vi "Device.vi"(8 "error in (no error)":errorcluster, 11 "Node Ptr":T1 format="%.0x") -> (0 "error out":errorcluster)   [LabVIEW 2013]
uses:
  <vilib>/NI Veristand/Custom Device API/Custom Device Item Ref.ctl
  <vilib>/NI Veristand/Custom Device API/Custom Device API.lvlib
panel:
  in  "Header":cluster{"Section Name":string}={"Section Name"="Custom Device Item Settings"}
  in  "Description":string
  in  "Name":string
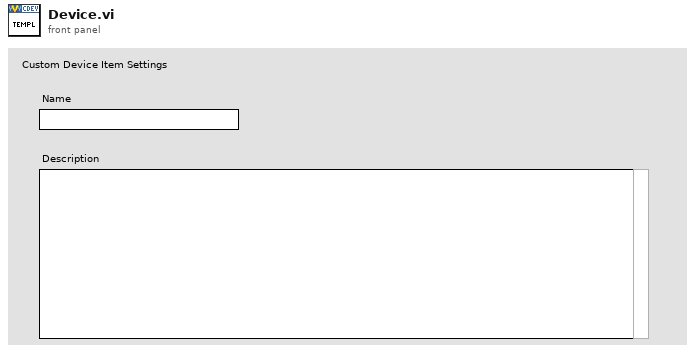
[diagram p1: front panel]
types:
  T1 = typedef "Custom Device API.lvlib/Custom Device Item Ref.ctl" = u64
  T2 = typedef "Custom Device API.lvlib/Custom Device Item Info.ctl" = cluster{"Name":string, "Is Channel":bool, "GUID":string, "Is Waveform":bool}
  T3 = typedef "Custom Device API.lvlib/Custom Device Commands.ctl" = enum16{"Default", "Item renamed", "Shutdown", "Dynamic button pressed"}
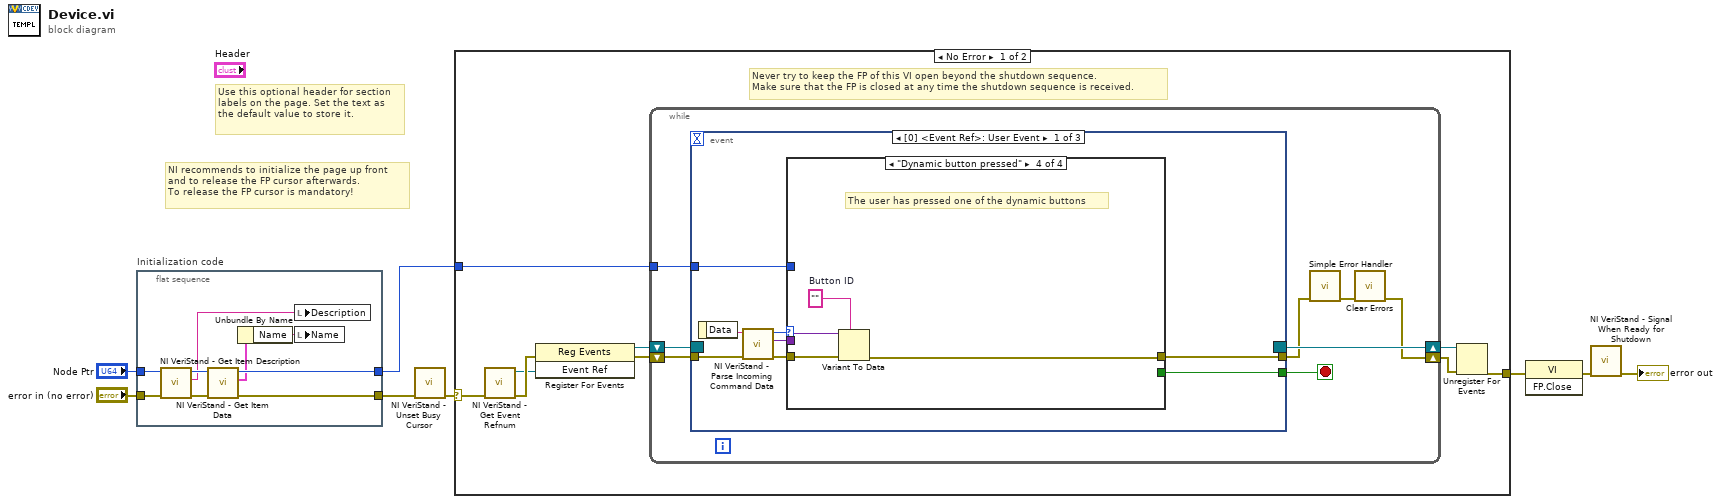
[diagram p0: block diagram]
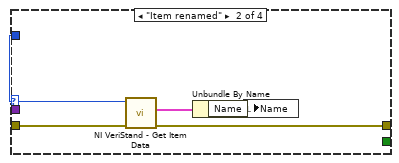
[diagram p3: hidden frame]
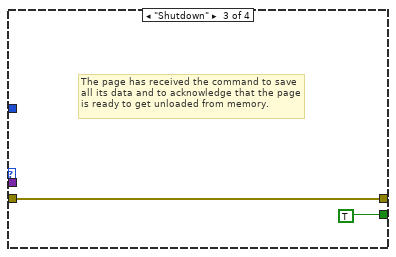
[diagram p4: hidden frame]
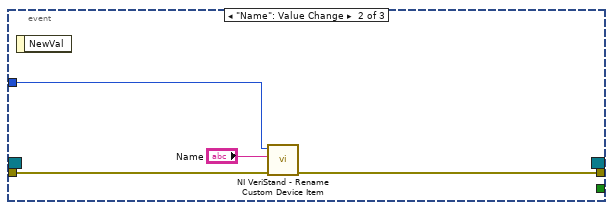
[diagram p5: hidden frame]
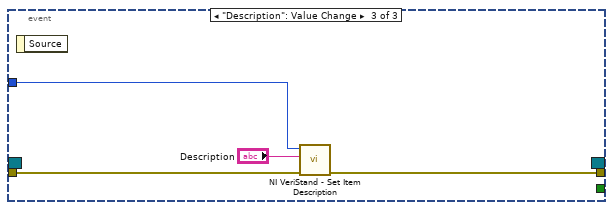
[diagram p6: hidden frame]
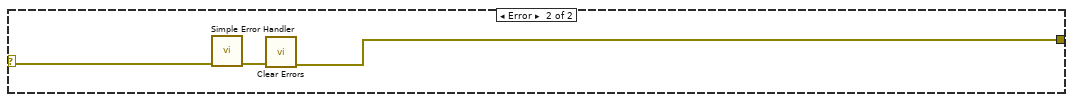
[diagram p7: hidden frame]
diagram:
  # "Use this optional header for section labels on the page. Set the text as the default value to store it."
  # "NI recommends to initialize the page up front\nand to release the FP cursor afterwards.\nTo release the FP cursor is mandatory!"
  n1 = flat-sequence "Initialization code" {
    tunnel: "error in (no error)" -> [w15]
    tunnel: "Node Ptr" -> [w14]
    tunnel: [w9] -> w4
    tunnel: [w17] -> w1
    frame #0 {
      n2 = call <vilib>:"NI VeriStand - Get Item Description.vi"("error in (no error)"=w15, "Item Ref in"=w14) -> ("error out"=w12:errorcluster, "Description"=w13:string, "Item Ref out"=w16:T1)  [unwired: 7 out]
      n3 = call <vilib>:"NI VeriStand - Get Item Data.vi"("error in (no error)"=w12, "Item Ref in"=w16) -> ("error out"=w9:errorcluster, "Item Info"=w11:T2, "Item Ref out"=w17:T1)  [unwired: 7 out]
      n4 = Unbundle By Name(w11) -> ("Name"=w10:string)
      n5 = local write "Description"(w13) -> ()
      n6 = local write "Name"(w10) -> ()
    }
  }
  n7 = call <vilib>:"NI VeriStand - Unset Busy Cursor.vi"("error in (no error)"=w4) -> ("error out"=w3:errorcluster)  [unwired: 10 out]
  n8 = case shown="No Error" w3 {
    selector: w3 -> [w18 w65]
    tunnel: [w23 w63] -> w8
    tunnel: w1 -> [w19 _]
    frame No Error {
      # "Never try to keep the FP of this VI open beyond the shutdown sequence.\nMake sure that the FP is closed at any time the shutdown sequence is received."
      n9 = call <vilib>:"NI VeriStand - Get Event Refnum.vi"("error in (no error)"=w18) -> ("error out"=w26:errorcluster, "Event Ref"=w22:refnum<user-event>)  [unwired: 9 out]
      n10 = register-events(error in=w26, w22) -> (reference out=w20:refnum<event-registration>, error out=w21:errorcluster)  [unwired: 1 in]
      n11 = while {
        tunnel: w19 -> [w30]
        shift-right: [w27] -> w24
        shift-left: w21 -> [w33]
        shift-right: [w34] -> w25
        shift-left: w20 -> [w32]
        stop <- w31 stop-if-true
        n12 = event shown="[0] <Event Ref>: User Event" {
          selector: w32 -> [_ _ _]
          dyn-events: [_ _ _] -> w34
          timeout: _ -> [_ _ _]
          tunnel: w33 -> [w42 w58 w61]
          tunnel: [w38 _ _] -> w31
          tunnel: [w37 w57 w60] -> w29
          tunnel: w30 -> [w36 w56 w62]
          event User Event {
            n13 = event-data() -> ("Data"=w41:string)  [unwired: 1 out]
            n14 = call <vilib>:"NI VeriStand - Parse Incoming Command Data.vi"("error in (no error)"=w42, "Incoming data"=w41) -> ("error out"=w40:errorcluster, "Outgoing data"=w35:variant, "Action"=w39:T3)  [unwired: 7 out]
            n15 = case shown="\"Dynamic button pressed\"" w39 {
              tunnel: w40 -> [w43 w48 w49 w54]
              tunnel: [_ _ TRUE _] -> w38
              tunnel: [w43 w45 w49 w51] -> w37
              tunnel: w36 -> [_ w47 _ _]
              tunnel: w35 -> [_ _ _ w53]
              frame "Default", Default {
              }
              frame "Item renamed" {
                n16 = call <vilib>:"NI VeriStand - Get Item Data.vi"("error in (no error)"=w48, "Item Ref in"=w47) -> ("error out"=w45:errorcluster, "Item Info"=w46:T2)  [unwired: 8 out]
                n17 = Unbundle By Name(w46) -> ("Name"=w44:string)
                n18 = local write "Name"(w44) -> ()
              }
              frame "Shutdown" {
                # "The page has received the command to save all its data and to acknowledge that the page is ready to get unloaded from memory."
              }
              frame "Dynamic button pressed" {
                w52 = ""  # Button ID
                # "The user has pressed one of the dynamic buttons"
                n19 = Variant To Data(error in=w54, type=w52, Variant=w53) -> (error out=w51:errorcluster)  [unwired: 1 out]
              }
            }
          }
          event "Name": Value Change {
            n20 = event-data() -> ()  [unwired: 2 out]
            n21 = call <vilib>:"NI VeriStand - Rename Custom Device Item.vi"("error in (no error)"=w58, "New Name"="Name", "Item Ref in"=w56) -> ("error out"=w57:errorcluster)  [unwired: 1 in, 7 out]
          }
          event "Description": Value Change {
            n22 = event-data() -> ()  [unwired: 2 out]
            n23 = call <vilib>:"NI VeriStand - Set Item Description.vi"("error in (no error)"=w61, "Description"="Description", "Item Ref in"=w62) -> ("error out"=w60:errorcluster)  [unwired: 8 out]
          }
        }
        n24 = call <vilib>:"Simple Error Handler.vi"("error in (no error)"=w29) -> ("error out"=w28:errorcluster)  [unwired: 1 in, 7 out]
        n25 = call <vilib>:"Clear Errors.vi"("error in (no error)"=w28) -> ("error out"=w27:errorcluster)  [unwired: 6 out]
      }
      n26 = Unregister For Events(event registration refnum=w25, error in=w24) -> (error out=w23:errorcluster)
    }
    frame Error {
      n27 = call <vilib>:"Simple Error Handler.vi"("error in (no error)"=w65) -> ("error out"=w64:errorcluster)  [unwired: 1 in, 7 out]
      n28 = call <vilib>:"Clear Errors.vi"("error in (no error)"=w64) -> ("error out"=w63:errorcluster)  [unwired: 6 out]
    }
  }
  n29 = invoke class="VI" method="FP.Close"(error in=w8) -> (error out=w7:errorcluster)  [unwired: 2 in, 2 out]
  n30 = call <vilib>:"NI VeriStand - Signal When Ready for Shutdown.vi"("error in (no error)"=w7) -> ("error out"=→"error out":errorcluster)  [unwired: 10 out]
